vi "CMO.vi"(0 "System no.":i32=1 min=1 max=4 step=1, 2 "Axes to set":string[](array[string]), 3 "Control Mode":i32[](array[numeric]), 5 "error in":errorcluster) -> (14 "Controller error":bool, 19 "error out":errorcluster)   [LabVIEW 2020]
doc: "Sets the control mode and checks for error. Controller error is TRUE if selected system reports error code unequal to 0."
panel:
  # "Sets the control mode and checks for error."
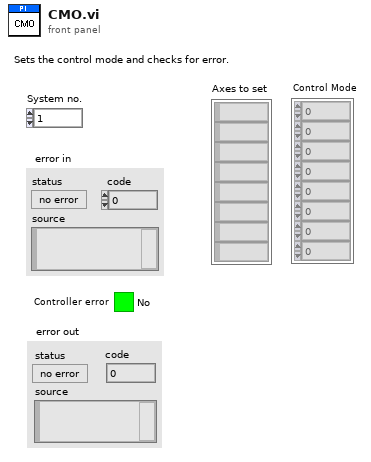
[diagram p1: front panel]
types:
  T1 = enum16{"Disable error check", "Force error check", "Use global settings"}
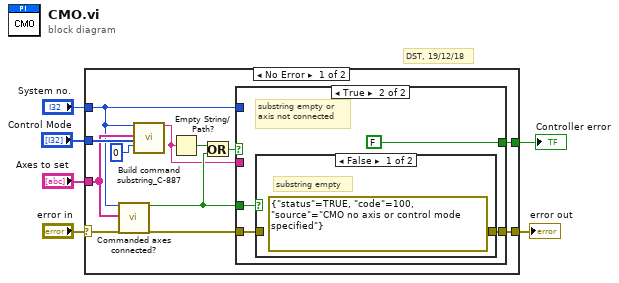
[diagram p0: block diagram]
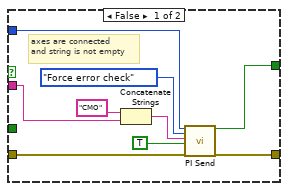
[diagram p2: hidden frame]
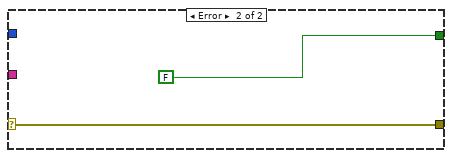
[diagram p4: hidden frame]
diagram:
  # "DST, 19/12/18"
  n1 = case shown="No Error" "error in" {
    selector: "error in" -> [w12 w35]
    tunnel: [w18 w35] -> w6
    tunnel: "Control Mode" -> [w17 _]
    tunnel: "System no." -> [w14 _]
    tunnel: "Axes to set" -> [w15 _]
    tunnel: [w7 FALSE ("Controller error")] -> w1
    frame No Error {
      n2 = call "Commanded axes connected?.vi"("System no."=w14, "Commanded axes"=w15, "error in"=w12) -> ("Controller error"=w10:bool, "error out"=w16:errorcluster)  [unwired: 1 in, 14 out]
      n3 = call "Build command substring_C-887.vi"("System no."=w14, "Affected axes"=w15, "Parameters"=w17, "No. of digits"=i16 0) -> ("Command substring"=w8:string)  [unwired: 3 in, 12 out]
      n4 = Empty String/Path?(string/path=w8) -> (empty?=w9:bool)
      n5 = Or(x=w9, y=w10) -> (x .or. y?=w11:bool)
      n6 = case shown="True" w11 {
        tunnel: w8 -> [w26 _]
        tunnel: [w20 w31] -> w18
        tunnel: w16 -> [w23 w29]
        tunnel: w10 -> [_ w30]
        tunnel: w14 -> [w22 _]
        tunnel: [w19 FALSE ("Controller error")] -> w7
        frame False {
          # "axes are connected\nand string is not empty"
          n7 = Concatenate Strings("CMO", w26) -> (w24:string)
          n8 = call "PI Send.vi"("System no."=w22, "Error check settings"=T1."Force error check", "String to send"=w24, "Attach termination char.?"=TRUE ("Attach Linefeed?"), "error in"=w23) -> ("Controller error"=w19:bool, "error out"=w20:errorcluster)  [unwired: 1 in, 12 out]
        }
        frame True {
          # "substring empty or \naxis not connected"
          n9 = case shown="False" w30 {
            tunnel: [errorcluster {"status"=TRUE, "code"=100, "source"="CMO no axis or control mode specified"} ("error out") w33] -> w31
            tunnel: w29 -> [_ w33]
            frame False {
              # "substring empty"
            }
            frame True {
              # "commanded axis\nnot connected"
            }
          }
        }
      }
    }
    frame Error {
    }
  }
  "error out" <- w6
  "Controller error" <- w1
